vi "Scan Page find supports.vi"(11 "Block Array":i32[][][](array[numeric])) -> (3 "Support Map":map{i32, set{i32}}(c390))   [LabVIEW 2023]
uses:
  <vilib>/Utility/miscctls.llb/LVMapReplaceAction.ctl
panel:
  out "Numeric":i32
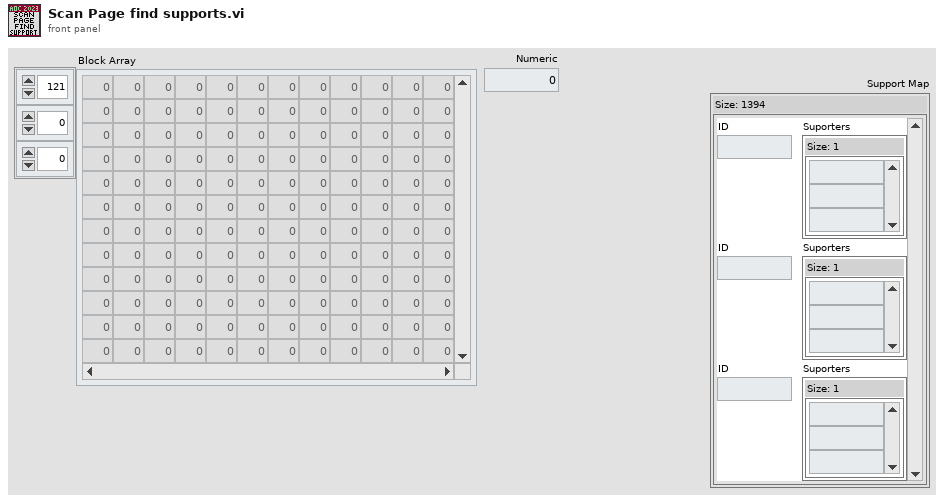
[diagram p1: front panel]
types:
  T1 = typedef "LVMapReplaceAction.ctl" = enum32{"Modify Entry only if found", "Add or Modify Entry", "Delete Entry"}
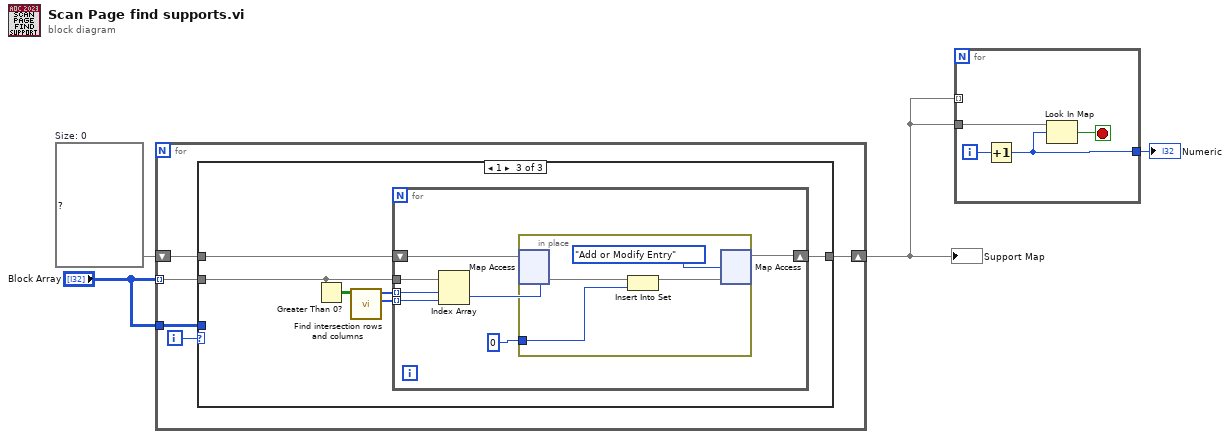
[diagram p0: block diagram]
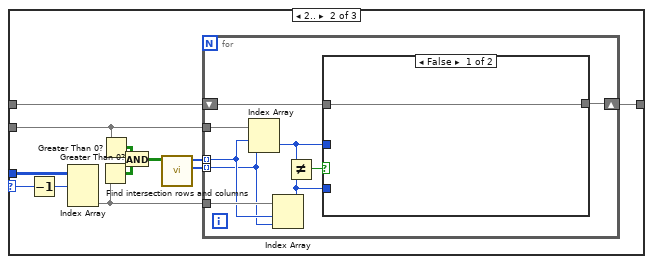
[diagram p3: hidden frame]
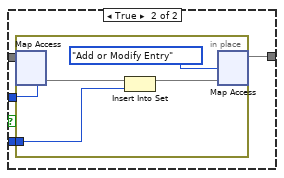
[diagram p4: hidden frame]
diagram:
  w4 = map{i32, set{i32}} {}  # Size: 0
  n1 = for {
    tunnel: "Block Array" -> [w9]
    tunnel: "Block Array" -> [w7] mode=indexing
    shift-right: [w5] -> w1
    shift-left: w4 -> [w6]
    i -> [w8]
    n2 = case shown="1" w8 {
      selector: w8 -> [_ w18 _]
      tunnel: w9 -> [_ w19 _]
      tunnel: w7 -> [_ w17 w46]
      tunnel: w6 -> [w10 w14 w45]
      tunnel: [w10 w11 w42] -> w5
      frame ..0 {
      }
      frame 2.. {
        n3 = Decrement(x=w18) -> (x-1=w16:i32)
        n4 = Index Array(array=w19, index (dim 0)=w16) -> (element=w15:i32[][])  [unwired: 2 in]
        n5 = Greater Than 0?(x=w15) -> (x > 0?=w22:bool[][])
        n6 = Greater Than 0?(x=w17) -> (x > 0?=w21:bool[][])
        n7 = And(x=w21, y=w22) -> (x .and. y?=w20:bool[][])
        n8 = call "Find intersection rows and columns.vi"("Page intersection array"=w20) -> ("Columns"=w12:i32[], "Rows"=w13:i32[])  [unwired: 9 in]
        n9 = for {
          tunnel: w13 -> [w29] mode=indexing
          tunnel: w12 -> [w28] mode=indexing
          tunnel: w17 -> [w31]
          tunnel: w15 -> [w30]
          shift-right: [w23] -> w11
          shift-left: w14 -> [w26]
          n10 = Index Array(array=w31, index (row)=w29, index (col)=w28) -> (element=w24:i32)
          n11 = Index Array(array=w30, index (row)=w29, index (col)=w28) -> (element=w25:i32)
          n12 = Not Equal?(x=w24, y=w25) -> (x != y?=w27:bool)
          n13 = case shown="False" w27 {
            tunnel: w26 -> [w32 w36]
            tunnel: w25 -> [_ w33]
            tunnel: w24 -> [_ w34]
            tunnel: [w32 w35] -> w23
            frame False {
            }
            frame True {
              n14 = in-place {
                in-place-border: w33 -> [w38]
                n15 = in-place-map #1(w36, w34) -> (w40:set{i32})  [unwired: 1 in, 1 out]
                n16 = Insert Into Set(10:w38, 11:w40) -> (3:w39:set{i32})  [unwired: 1 out]
                n17 = in-place-map #1(w39, LVMapReplaceAction."Add or Modify Entry" ("action")) -> (w35:map{i32, set{i32}})  [unwired: 2 out]
              }
            }
          }
        }
      }
      frame 1 {
        n18 = Greater Than 0?(x=w46) -> (x > 0?=w41:bool[][])
        n19 = call "Find intersection rows and columns.vi"("Page intersection array"=w41) -> ("Columns"=w43:i32[], "Rows"=w44:i32[])  [unwired: 9 in]
        n20 = for {
          tunnel: w44 -> [w52] mode=indexing
          tunnel: w43 -> [w51] mode=indexing
          tunnel: w46 -> [w53]
          shift-right: [w48] -> w42
          shift-left: w45 -> [w50]
          n21 = Index Array(array=w53, index (row)=w52, index (col)=w51) -> (element=w49:i32)
          n22 = in-place {
            in-place-border: 0 ("max value") -> [w55]
            n23 = in-place-map #2(w50, w49) -> (w57:set{i32})  [unwired: 1 in, 1 out]
            n24 = Insert Into Set(10:w55, 11:w57) -> (3:w56:set{i32})  [unwired: 1 out]
            n25 = in-place-map #2(w56, LVMapReplaceAction."Add or Modify Entry" ("action")) -> (w48:map{i32, set{i32}})  [unwired: 2 out]
          }
        }
      }
    }
  }
  "Support Map" <- w1
  n26 = for {
    tunnel: w1 -> [w61]
    tunnel: [w58] -> w2
    tunnel: w1 -> [_] mode=indexing
    i -> [w60]
    stop <- w59 stop-if-true
    n27 = Increment(x=w60) -> (x+1=w58:i32)
    n28 = Look In Map(map=w61, key=w58) -> (key not found?=w59:bool)  [unwired: 1 in, 1 out]
  }
  "Numeric" <- w2
